vi "Find BuildSpec.vi"(8 "Error In":errorcluster, 9 "Build Spec Name in":string, 10 "Target Name in":string, 11 "Project Sync Tools in":refnum<class "Project Sync Tools.lvclass">) -> (0 "Error Out":errorcluster, 1 "Found ?":bool, 2 "Build Spec out":T1, 3 "Project Sync Tools out":refnum<class "Project Sync Tools.lvclass">)   [LabVIEW 2019, in "Project Sync Tools.lvclass"]
uses:
  Project Sync Tools.lvclass
  TypeDefs/BuildSpec Parameters.ctl
  Project Sync Tools.lvclass/Project Sync Tools.ctl
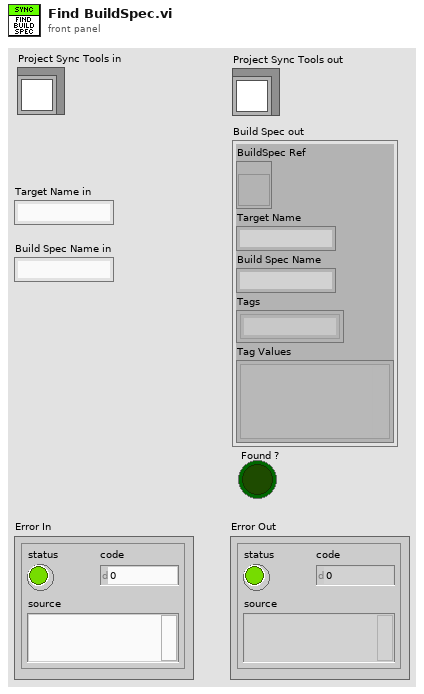
[diagram p1: front panel]
types:
  T1 = typedef "Project Sync Tools.lvclass/BuildSpec Parameters.ctl" = cluster{"BuildSpec Ref":refnum<vi>, "Target Name":string, "Build Spec Name":string, "Tags":string[], "Tag Values":variant[]}
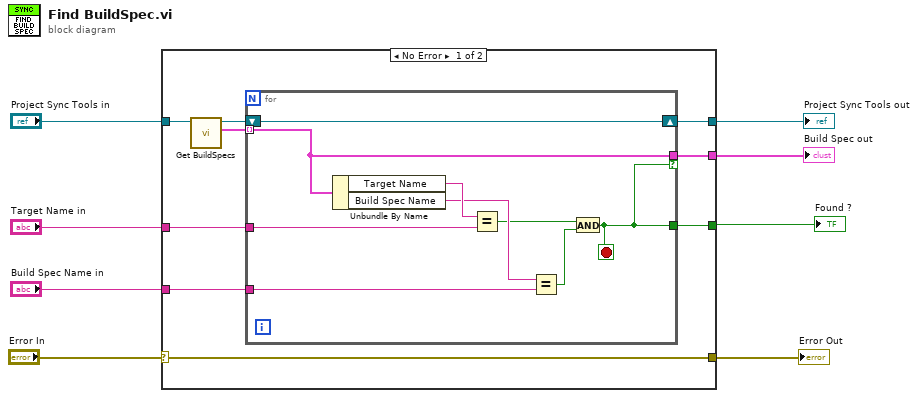
[diagram p0: block diagram]
diagram:
  n1 = case shown="No Error" "Error In" {
    selector: "Error In" -> [w10 w27]
    tunnel: [w17 w28] -> w8
    tunnel: "Project Sync Tools in" -> [w15 w28]
    tunnel: "Build Spec Name in" -> [w14 _]
    tunnel: "Target Name in" -> [w13 _]
    tunnel: [w11 _] -> w4
    tunnel: [w10 w27] -> w2
    tunnel: [w9 _] -> w1
    frame No Error {
      n2 = call "Get BuildSpecs.vi"("Project Sync Tools in"=w15) -> ("BuildSpecs"=w12:T1[], "Project Sync Tools out"=w16:refnum<class "Project Sync Tools.lvclass">)  [unwired: 9 in]
      n3 = for {
        tunnel: w12 -> [w19] mode=indexing
        tunnel: w13 -> [w25]
        tunnel: w14 -> [w23]
        shift-right: [w22] -> w17
        shift-left: w16 -> [w22]
        tunnel: [w18] -> w9
        tunnel: [w19] -> w11 if=w18
        stop <- w18 stop-if-true
        n4 = Unbundle By Name(w19) -> ("Target Name"=w26:string, "Build Spec Name"=w24:string)
        n5 = Equal?(x=w26, y=w25) -> (x = y?=w21:bool)
        n6 = Equal?(x=w24, y=w23) -> (x = y?=w20:bool)
        n7 = And(x=w21, y=w20) -> (x .and. y?=w18:bool)
      }
    }
    frame Error {
    }
  }
  "Project Sync Tools out" <- w8
  "Build Spec out" <- w4
  "Error Out" <- w2
  "Found ?" <- w1
